vi "Message encoder.vi"(8 "error in (no error)":errorcluster, 10 "Data":variant, 11 "TCP Text Writer in":refnum<class "TCP Text Writer.lvclass">) -> (0 "error out":errorcluster, 2 "Message encoded":string, 3 "TCP Text Writer out":refnum<class "TCP Text Writer.lvclass">)   [LabVIEW 2026, in "TALOS.lvlib" / "TCP Text Writer.lvlib" / "TCP Text Writer.lvclass"]
uses:
  TCP Text Writer.lvclass
  Ancestor/Ancestor/Ancestor.lvclass/Ancestor.ctl
  <vilib>/AdvancedString/1D String Array to Delimited String (string).vi
  Support VIs/Generate Error.vi
  FGV/Error Memory/Get Error Description.vi
  Support VIs/Get PC name.vi
  Ancestor/Ancestor/Read ID.vi
  Support VIs/Get Class Name.vi
  FGV/Error Memory/Error Memory Core.vi
  <vilib>/AdvancedString/Delimited String to 1D String Array.vi
  <vilib>/AdvancedString/Delimited String to 1D String Array (string).vi
  Support VIs/Circus Root Path.vi
  FGV/Error Memory/Error Crt Lvl checker.vi
  FGV/Error Memory/Error Memory Core.vi/40c8088d-b597-4017-91af-faa98e00292e.vi
  FGV/Error Memory/Error Memory Core.vi/d4a3ab98-063c-4e44-b43d-fbdcfe6c2be2.vi
  Support VIs/Global Constants.vi
  Support VIs/Global Memory.vi
  <vilib>/Utility/LVClass/Get LV Class Name.vi
  Support VIs/Is in Packed Library.vi
  Support VIs/TALOS Root path.vi
  Support VIs/Read CSV worksheet.vi
  <vilib>/Utility/error.llb/General Error Handler.vi
  Support VIs/Error Log.vi
  Ancestor/Ancestor/Ancestor.lvclass
  <vilib>/Comparison/Equal/Equal Functor/Equal Functor.lvclass
  TALOS.lvlib
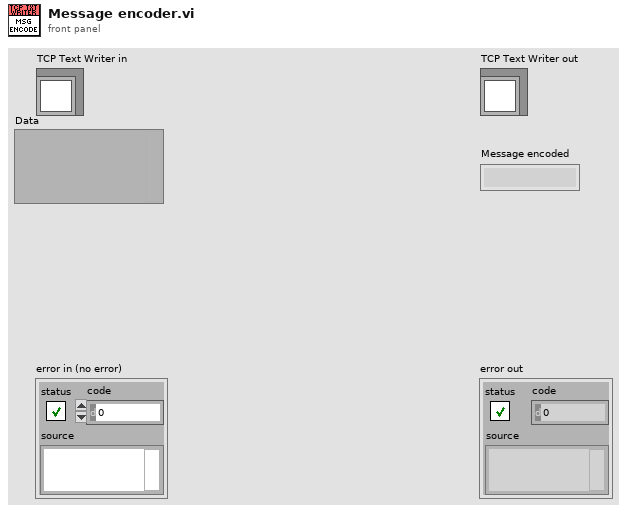
[diagram p1: front panel]
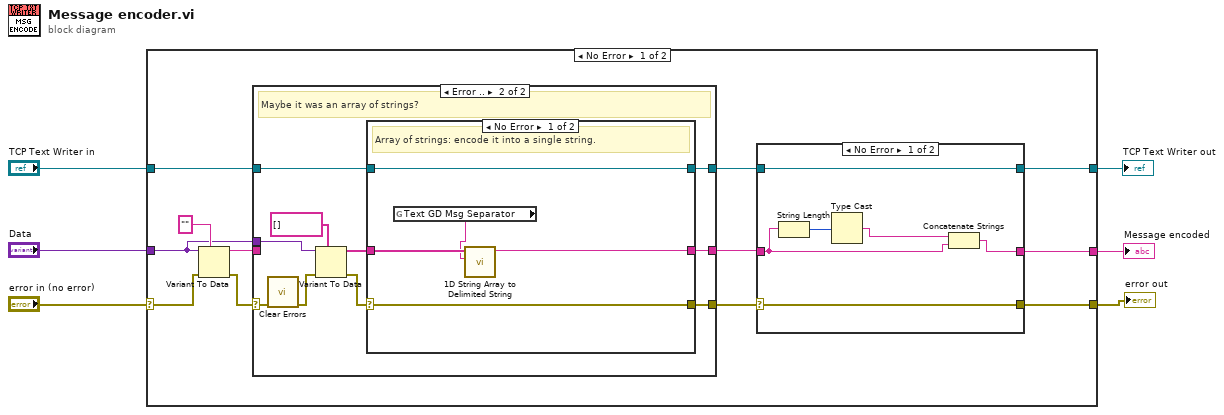
[diagram p0: block diagram]
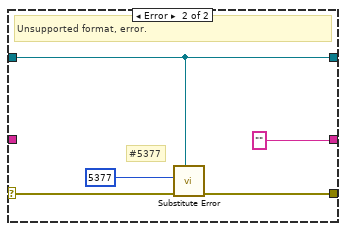
[diagram p3: hidden frame]
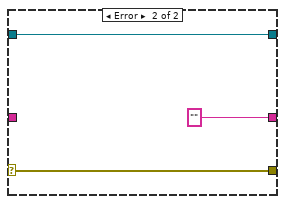
[diagram p4: hidden frame]
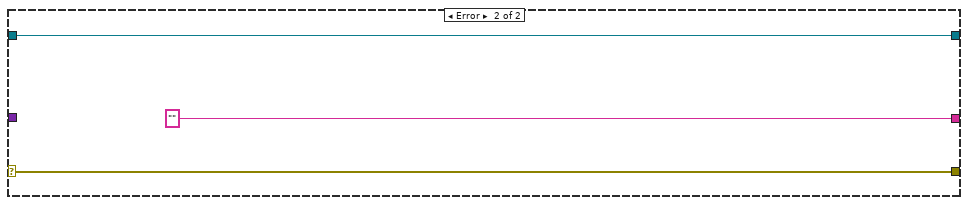
[diagram p5: hidden frame]
diagram:
  n1 = case shown="No Error" "error in (no error)" {
    selector: "error in (no error)" -> [w14 w53]
    tunnel: [w16 w53] -> w1
    tunnel: [w18 w52] -> w3
    tunnel: "TCP Text Writer in" -> [w8 w52]
    tunnel: [w17 "" ("data string")] -> w2
    tunnel: "Data" -> [w7 _]
    frame No Error {
      n2 = Variant To Data(error in=w14, type="", Variant=w7) -> (data=w11:string, error out=w12:errorcluster)
      n3 = case shown="Error .." w12 {
        selector: w12 -> [w21 w23]
        tunnel: [w21 w29] -> w13
        tunnel: w11 -> [w20 _]
        tunnel: [w20 w26] -> w10
        tunnel: [w19 w25] -> w9
        tunnel: w8 -> [w19 w24]
        tunnel: w7 -> [_ w31]
        frame No Error {
          # "It was simply a string, send it out."
        }
        frame Error {
          # "Maybe it was an array of strings?"
          n4 = call <vilib>:"Clear Errors.vi"("error in (no error)"=w23) -> ("error out"=w22:errorcluster)  [unwired: 5 in, 1 out]
          n5 = Variant To Data(error in=w22, type=string[] [], Variant=w31) -> (data=w27:string[], error out=w28:errorcluster)
          n6 = case shown="No Error" w28 {
            selector: w28 -> [w36 w40]
            tunnel: [w36 w38] -> w29
            tunnel: w27 -> [w35 _]
            tunnel: [w33 ""] -> w26
            tunnel: [w32 w37] -> w25
            tunnel: w24 -> [w32 w37]
            frame No Error {
              # "Array of strings: encode it into a single string."
              n7 = global read "Global Constants.vi" "Text GD Msg Separator"() -> (w34:string)
              n8 = call-poly <vilib>:"1D String Array to Delimited String.vi"("delimiter"=w34, "string array"=w35) -> ("delimited string"=w33:string)  [unwired: 9 in]
            }
            frame Error {
              # "#5377"
              # "Unsupported format, error."
              n9 = call "Substitute Error.vi"("LabVIEW Object"=w37, "error in (no error)"=w40, "Error Code"=5377) -> ("error out"=w38:errorcluster)  [unwired: 8 in]
            }
          }
        }
      }
      n10 = case shown="No Error" w13 {
        selector: w13 -> [w43 w49]
        tunnel: [w47 w50] -> w18
        tunnel: w9 -> [w47 w50]
        tunnel: w10 -> [w45 _]
        tunnel: [w44 ""] -> w17
        tunnel: [w43 w49] -> w16
        frame No Error {
          n11 = String Length(string=w45) -> (length=w42:i32)
          n12 = Type Cast(x=w42) -> (*(type *) &x=w46:string)  [unwired: 1 in]
          n13 = Concatenate Strings(w46, w45) -> (w44:string)
        }
        frame Error {
        }
      }
    }
    frame Error {
    }
  }
  "error out" <- w1
  "TCP Text Writer out" <- w3
  "Message encoded" <- w2
